vi "SP Range Check with Precision.vi"(8 "precision":i32=8, 9 "low":dbl format="%0.20f", 10 "x":dbl format="%0.20f", 11 "high":dbl format="%0.20f") -> (3 "range result":T1(ring))   [LabVIEW 2011]
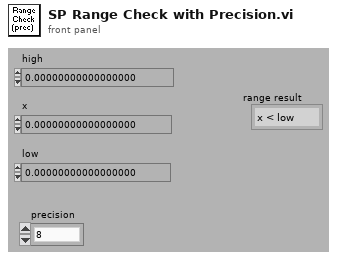
[diagram p1: front panel]
types:
  T1 = enum16{"x < low", "low <= x <= high", "x > high"}
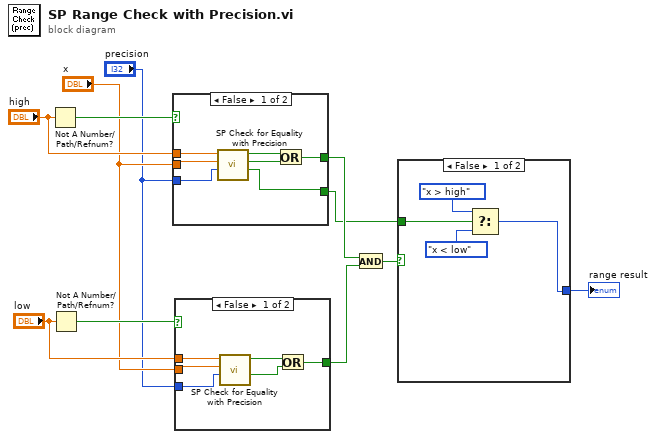
[diagram p0: block diagram]
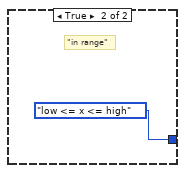
[diagram p2: hidden frame]
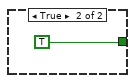
[diagram p3: hidden frame]
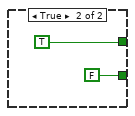
[diagram p4: hidden frame]
diagram:
  n1 = Not A Number/Path/Refnum?(number/path/refnum="high") -> (NaN/Path/Refnum?=w11:bool)
  n2 = Not A Number/Path/Refnum?(number/path/refnum="low") -> (NaN/Path/Refnum?=w8:bool)
  n3 = case shown="False" w11 {
    tunnel: "x" -> [w17 _]
    tunnel: "high" -> [w18 _]
    tunnel: [w14 TRUE] -> w9
    tunnel: "precision" -> [w13 _]
    tunnel: [w12 FALSE ("n1 < n2?")] -> w1
    frame False {
      n4 = call "SP Check for Equality with Precision.vi"("precision"=w13, "n2"=w17, "n1"=w18) -> ("n1 < n2?"=w12:bool, "n1 > n2?"=w15:bool, "equal (within precision)"=w16:bool)  [unwired: 6 out]
      n5 = Or(x=w16, y=w15) -> (x .or. y?=w14:bool)
    }
    frame True {
    }
  }
  n6 = case shown="False" w8 {
    tunnel: "x" -> [w25 _]
    tunnel: "low" -> [w26 _]
    tunnel: [w23 TRUE] -> w5
    tunnel: "precision" -> [w21 _]
    frame False {
      n7 = call "SP Check for Equality with Precision.vi"("precision"=w21, "n2"=w25, "n1"=w26) -> ("n1 < n2?"=w22:bool, "equal (within precision)"=w24:bool)  [unwired: 7 out]
      n8 = Or(x=w24, y=w22) -> (x .or. y?=w23:bool)
    }
    frame True {
    }
  }
  n9 = And(x=w9, y=w5) -> (x .and. y?=w3:bool)
  n10 = case shown="False" w3 {
    tunnel: [w30 T1."low <= x <= high" ("range result")] -> w2
    tunnel: w1 -> [w31 _]
    frame False {
      n11 = Select(t=T1."x > high" ("range result"), s=w31, f=T1."x < low" ("range result")) -> (s? t:f=w30:T1)
    }
    frame True {
      # "\"in range\""
    }
  }
  "range result" <- w2
